vi "Shutdown.vi"(8 "error in":errorcluster, 11 "device data model in":refnum<class "Device Data Model.lvclass">) -> (0 "error out":errorcluster)   [LabVIEW 2014, in "MyLib.lvlib" / "Device Data Model.lvclass"]
doc: "This VI is responsible for deleting the device data model."
uses:
  Device Data Model.lvclass
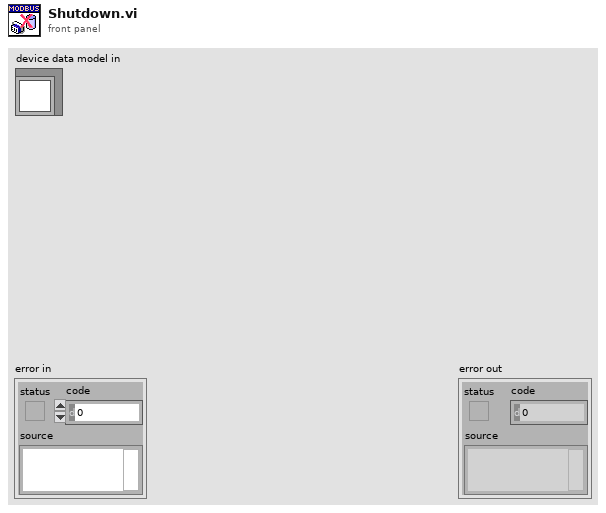
[diagram p1: front panel]
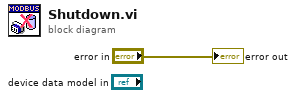
[diagram p0: block diagram]
diagram:
  "error out" <- "error in"
